vi "Simulate Keysight 34401a.vi"() -> ()   [LabVIEW 2021, in "Keysight_34401A-DMM.lvclass"]
uses:
  Keysight_34401A-DMM.lvclass
  <vilib>/Utility/config.llb/Read Key (String).vi
  <vilib>/Utility/config.llb/NI_LVConfig.lvlib
panel:
  in  "stop":bool
  out "error out":errorcluster
  in  "error in (no error)":errorcluster
  in  "VISA resource name":refnum<visa-resource-name>
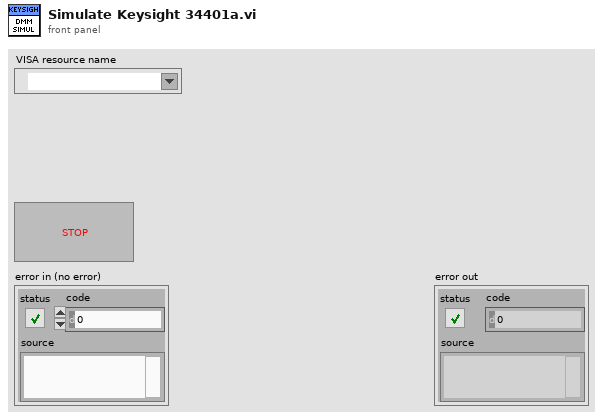
[diagram p1: front panel]
types:
  T1 = typedef "NI_LVConfig.lvlib/Config Data RefNum.ctl" = refnum<k1>
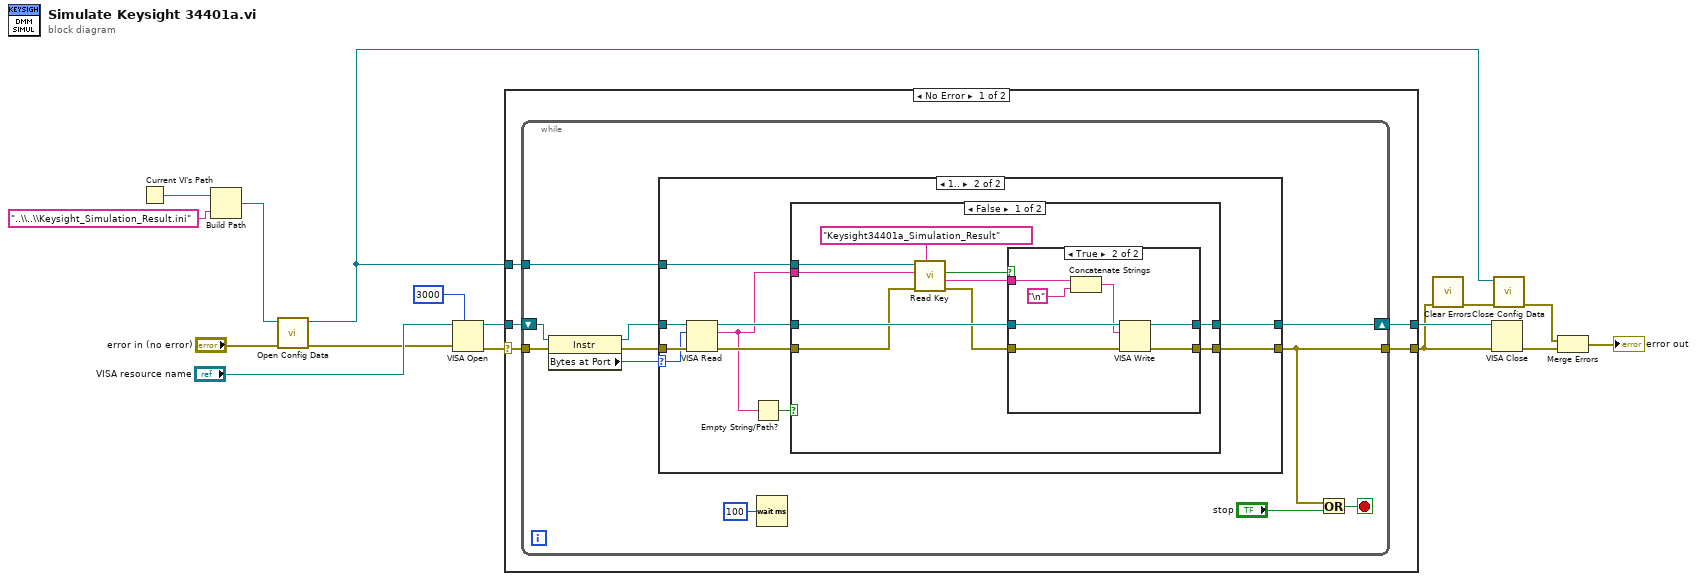
[diagram p0: block diagram]
diagram:
  n1 = Current VI's Path() -> (path=w9:path)
  n2 = Build Path(base path=w9, name or relative path="..\\..\\Keysight_Simulation_Result.ini" ("write buffer")) -> (appended path=w6:path)
  n3 = call <vilib>:"Open Config Data.vi"("error in (no error)"="error in (no error)", "configuration file path"=w6) -> ("error out"=w7:errorcluster, "refnum"=w5:T1)  [unwired: 7 in, 1 out]
  n4 = VISA Open(timeout (0)=u32 3000 ("VISA Open timeout (0)"), error in (no error)=w7, VISA resource name="VISA resource name") -> (VISA resource name=w13:refnum<visa-resource-name>, error out=w14:errorcluster)  [unwired: 2 in]
  n5 = case shown="No Error" w14 {
    selector: w14 -> [w21 w67]
    tunnel: w13 -> [w20 w66]
    tunnel: [w19 w67] -> w4
    tunnel: [w18 w66] -> w12
    tunnel: w5 -> [w17 _]
    frame No Error {
      n6 = while {
        tunnel: w21 -> [w32]
        tunnel: [w24] -> w19
        shift-right: [w27] -> w18
        shift-left: w20 -> [w29]
        tunnel: w17 -> [w23]
        stop <- w25 stop-if-true
        n7 = property class="Instr"(reference=w29, error in=w32) -> (reference out=w28:refnum<visa-resource-name>, error out=w30:errorcluster, "Bytes at Port"=w26:u32)
        n8 = case shown="1.." w26 {
          selector: w26 -> [_ w41]
          tunnel: w30 -> [w33 w44]
          tunnel: [w33 w40] -> w24
          tunnel: w28 -> [w34 w42]
          tunnel: [w34 w38] -> w27
          tunnel: w23 -> [_ w36]
          frame 0, Default {
          }
          frame 1.. {
            n9 = VISA Read(VISA resource name=w42, byte count=w41, error in (no error)=w44) -> (VISA resource name out=w39:refnum<visa-resource-name>, read buffer=w35:string, error out=w43:errorcluster)  [unwired: 1 out]
            n10 = Empty String/Path?(string/path=w35) -> (empty?=w37:bool)
            n11 = case shown="False" w37 {
              tunnel: w43 -> [w50 w64]
              tunnel: [w54 w64] -> w40
              tunnel: w39 -> [w53 w65]
              tunnel: [w52 w65] -> w38
              tunnel: w36 -> [w51 _]
              tunnel: w35 -> [w47 _]
              frame False {
                n12 = call-poly <vilib>:"Read Key.vi"("section"="Keysight34401a_Simulation_Result", "error in (no error)"=w50, "key"=w47, "refnum"=w51) -> ("error out"=w49:errorcluster, "value"=w45:string, "found?"=w46:bool)  [unwired: 4 in, 1 out]
                n13 = case shown="True" w46 {
                  tunnel: [w55 w63] -> w54
                  tunnel: w53 -> [w56 w62]
                  tunnel: [w56 w61] -> w52
                  tunnel: w49 -> [w55 w60]
                  tunnel: w45 -> [_ w59]
                  frame False {
                  }
                  frame True {
                    n14 = Concatenate Strings(w59, "\n") -> (w58:string)
                    n15 = VISA Write(VISA resource name=w62, write buffer=w58, error in (no error)=w60) -> (VISA resource name out=w61:refnum<visa-resource-name>, error out=w63:errorcluster)  [unwired: 1 out]
                  }
                }
              }
              frame True {
              }
            }
          }
        }
        n16 = Wait (ms)(milliseconds to wait=u32 100) -> ()  [unwired: 1 out]
        n17 = Or(x=w24, y="stop") -> (x .or. y?=w25:bool)
      }
    }
    frame Error {
    }
  }
  n18 = call <vilib>:"Clear Errors.vi"("error in (no error)"=w4) -> ("error out"=w3:errorcluster)  [unwired: 5 in, 1 out]
  n19 = VISA Close(VISA resource name=w12, error in (no error)=w4) -> (error out=w11:errorcluster)
  n20 = call <vilib>:"Close Config Data.vi"("error in (no error)"=w3, "refnum"=w5) -> ("error out"=w1:errorcluster)  [unwired: 8 in, 1 out]
  n21 = Merge Errors(w1, w11) -> (→"error out":errorcluster)
